vi "Meas Result Generate TWM Digitizer Correction - fit Gain Phase.vi"(7 "use time shift (true)":bool=TRUE, 9 "phase [rad]":dbl[](array[numeric]), 10 "gain [V/V]":dbl[](array[numeric]), 11 "f [Hz]":dbl[](array[numeric])) -> (0 "time shift [s]":dbl, 1 "DC gain":dbl, 2 "phase out [rad]":dbl[](array[numeric]), 3 "gain out [V/V]":dbl[](array[numeric]))   [LabVIEW 2013]
uses:
  <vilib>/Analysis/baseanly.llb/Mean (DBL).vi
  <vilib>/Analysis/NI_AALBase.lvlib
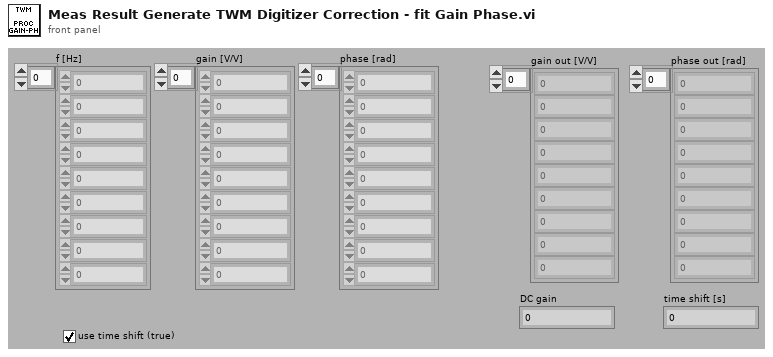
[diagram p1: front panel]
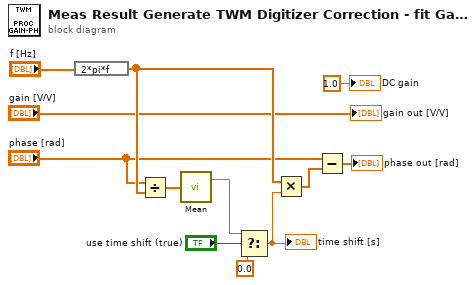
[diagram p0: block diagram]
diagram:
  n1 = expression code="2*pi*f"("f [Hz]") -> (w7:dbl[])
  n2 = Divide(x="phase [rad]", y=w7) -> (x/y=w11:dbl[])
  n3 = call-poly <vilib>:"Mean.vi"("X"=w11) -> ("mean"=w9:dbl)  [unwired: 1 out]
  n4 = Select(t=w9, s="use time shift (true)", f=0.0) -> (s? t:f=w3:dbl)
  "time shift [s]" <- w3
  n5 = Multiply(x=w7, y=w3) -> (x*y=w5:dbl[])
  n6 = Subtract(x="phase [rad]", y=w5) -> (x-y=→"phase out [rad]":dbl[])
  "gain out [V/V]" <- "gain [V/V]"
  "DC gain" <- 1.0 ("DC gain")
